vi "DiffDrivePoseEst2_Absolute_Example.vi"() -> ()   [LabVIEW 2019]
doc: "This WebSockets API example VI acts as a server for an incoming websockets connection. Receives/sends string data to the connected client."
uses:
  <vilib>/Rock Robotics/WPI/ThirdParty/JAS_Junk/TrajLib/Trajectory_Library.lvlib
  <vilib>/Rock Robotics/WPI/ThirdParty/JAS_Junk/TrajLib/TypeDef/FieldDisp_ElementPicture.ctl
  <vilib>/Rock Robotics/WPI/ThirdParty/JAS_Junk/TrajLib/TypeDef/TRANSLATION2D.ctl
  <vilib>/Rock Robotics/WPI/ThirdParty/JAS_Junk/TrajLib/TypeDef/ROTATION2D.ctl
  <vilib>/Rock Robotics/WPI/ThirdParty/JAS_Junk/TrajLib/TypeDef/POSE2D.ctl
panel:
  in  "Ramsette\nAuto":bool=TRUE
  out "Trajectory\nAtReference":bool
  out "ROBOT":T1
  in  "Tab Control":T2(tab)
  out "Field Picture":picture
  out "Right Motor Dmd":dbl format="%20.3f"
  out "Left Motor Dmd":dbl format="%20.3f"
  out "Gyro Heading (Deg)":dbl format="%20.3f"
  out "Left Motor Dist (Ft)":dbl format="%20.3f"
  out "Right Motor Dist (Ft)":dbl format="%20.3f"
  out "Left Motor Vel - PV (Ft/Sec)":dbl format="%20.3f"
  out "Right Motor Vel - PV (Ft/Sec)":dbl format="%20.3f"
  out "Odometry sim abs\n Pose SI":T3={"TRANSLATION"={"X"=1.0, "Y"=1.0}, "ROTATION"={"VALUE"=0.0, "COS"=1.0, "SIN"=0.0}} {"ROTATION"."SIN" format="%13.4f"; "ROTATION"."COS" format="%13.4f"; "ROTATION"."VALUE" format="%13.4f"; "TRANSLATION"."Y" format="%14.3f"; "TRANSLATION"."X" format="%14.3f"}
  out "Odom Abs Pose SI":T3 {"ROTATION"."SIN" format="%13.4f"; "ROTATION"."COS" format="%13.4f"; "ROTATION"."VALUE" format="%13.4f"; "TRANSLATION"."Y" format="%14.3f"; "TRANSLATION"."X" format="%14.3f"}
  out "Trajectory Error":T6(graph)
  in  "Follow Absolute\nTrajectory":bool
  in  "Spin Right":bool
  in  "Spin Left":bool
  in  "Reverse":bool
  in  "Forward":bool
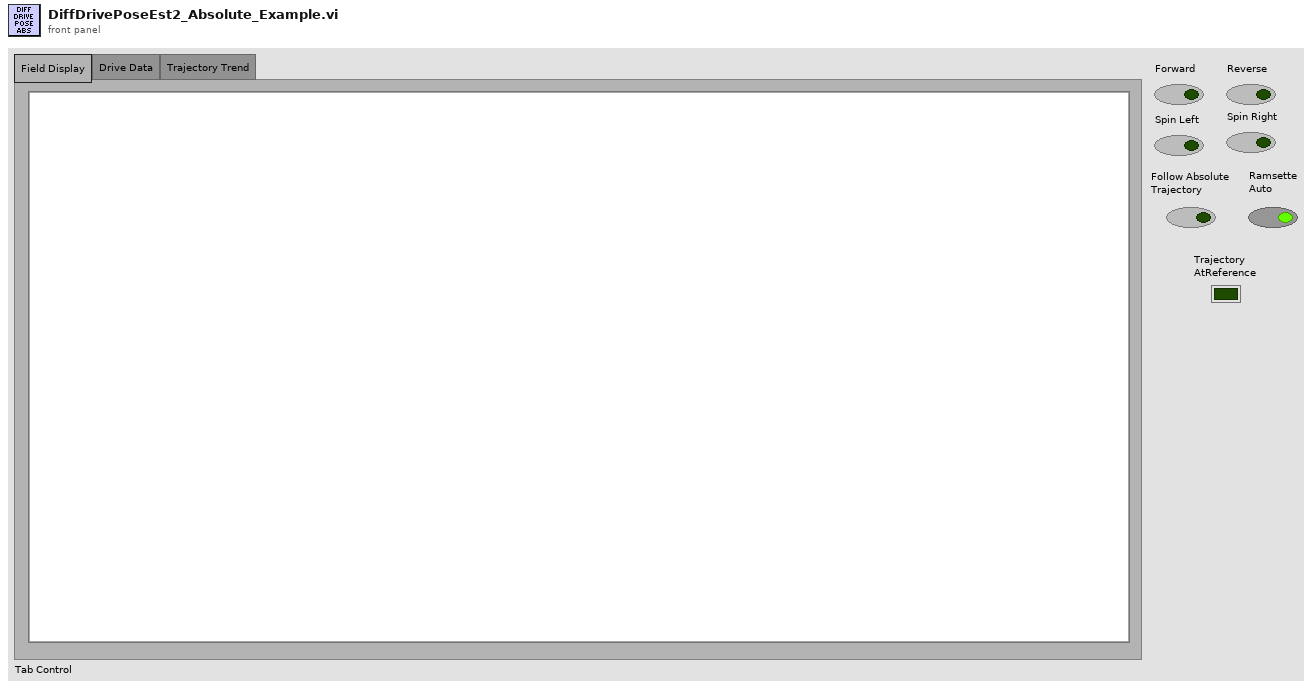
[diagram p1: front panel]
types:
  T1 = typedef "Trajectory_Library.lvlib/FieldDisp_ElementPicture.ctl" = picture
  T2 = enum32{"Field Display", "Drive Data", "Trajectory Trend"}
  T3 = typedef "Trajectory_Library.lvlib/POSE2D.ctl" = cluster{"TRANSLATION":T4, "ROTATION":T5}
  T4 = typedef "Trajectory_Library.lvlib/TRANSLATION2D.ctl" = cluster{"X":dbl, "Y":dbl}
  T5 = typedef "Trajectory_Library.lvlib/ROTATION2D.ctl" = cluster{"VALUE":dbl, "COS":dbl, "SIN":dbl}
  T6 = cluster{"Traj X Err Ft":dbl, "Traj Y Err Ft":dbl, "Traj Heading Err Deg":dbl, dbl}
  T7 = typedef "Trajectory_Library.lvlib/FieldDisp_FieldElement.ctl" = cluster{"ONE-8-bit pixmap":u8[][], "Two-Array":cdb[][], "Three-Numeric":i32, "Four-Numeric":i32, "Five-Numeric":cdb, "Six-colors":u32[], "Seven-new element/subarray":u32, "Left Poxel":dbl, "Top Pixel":dbl, "Width Pix/Ft":dbl, "Height Pix/Ft":dbl, "Element Picture Ref":refnum<vi>}
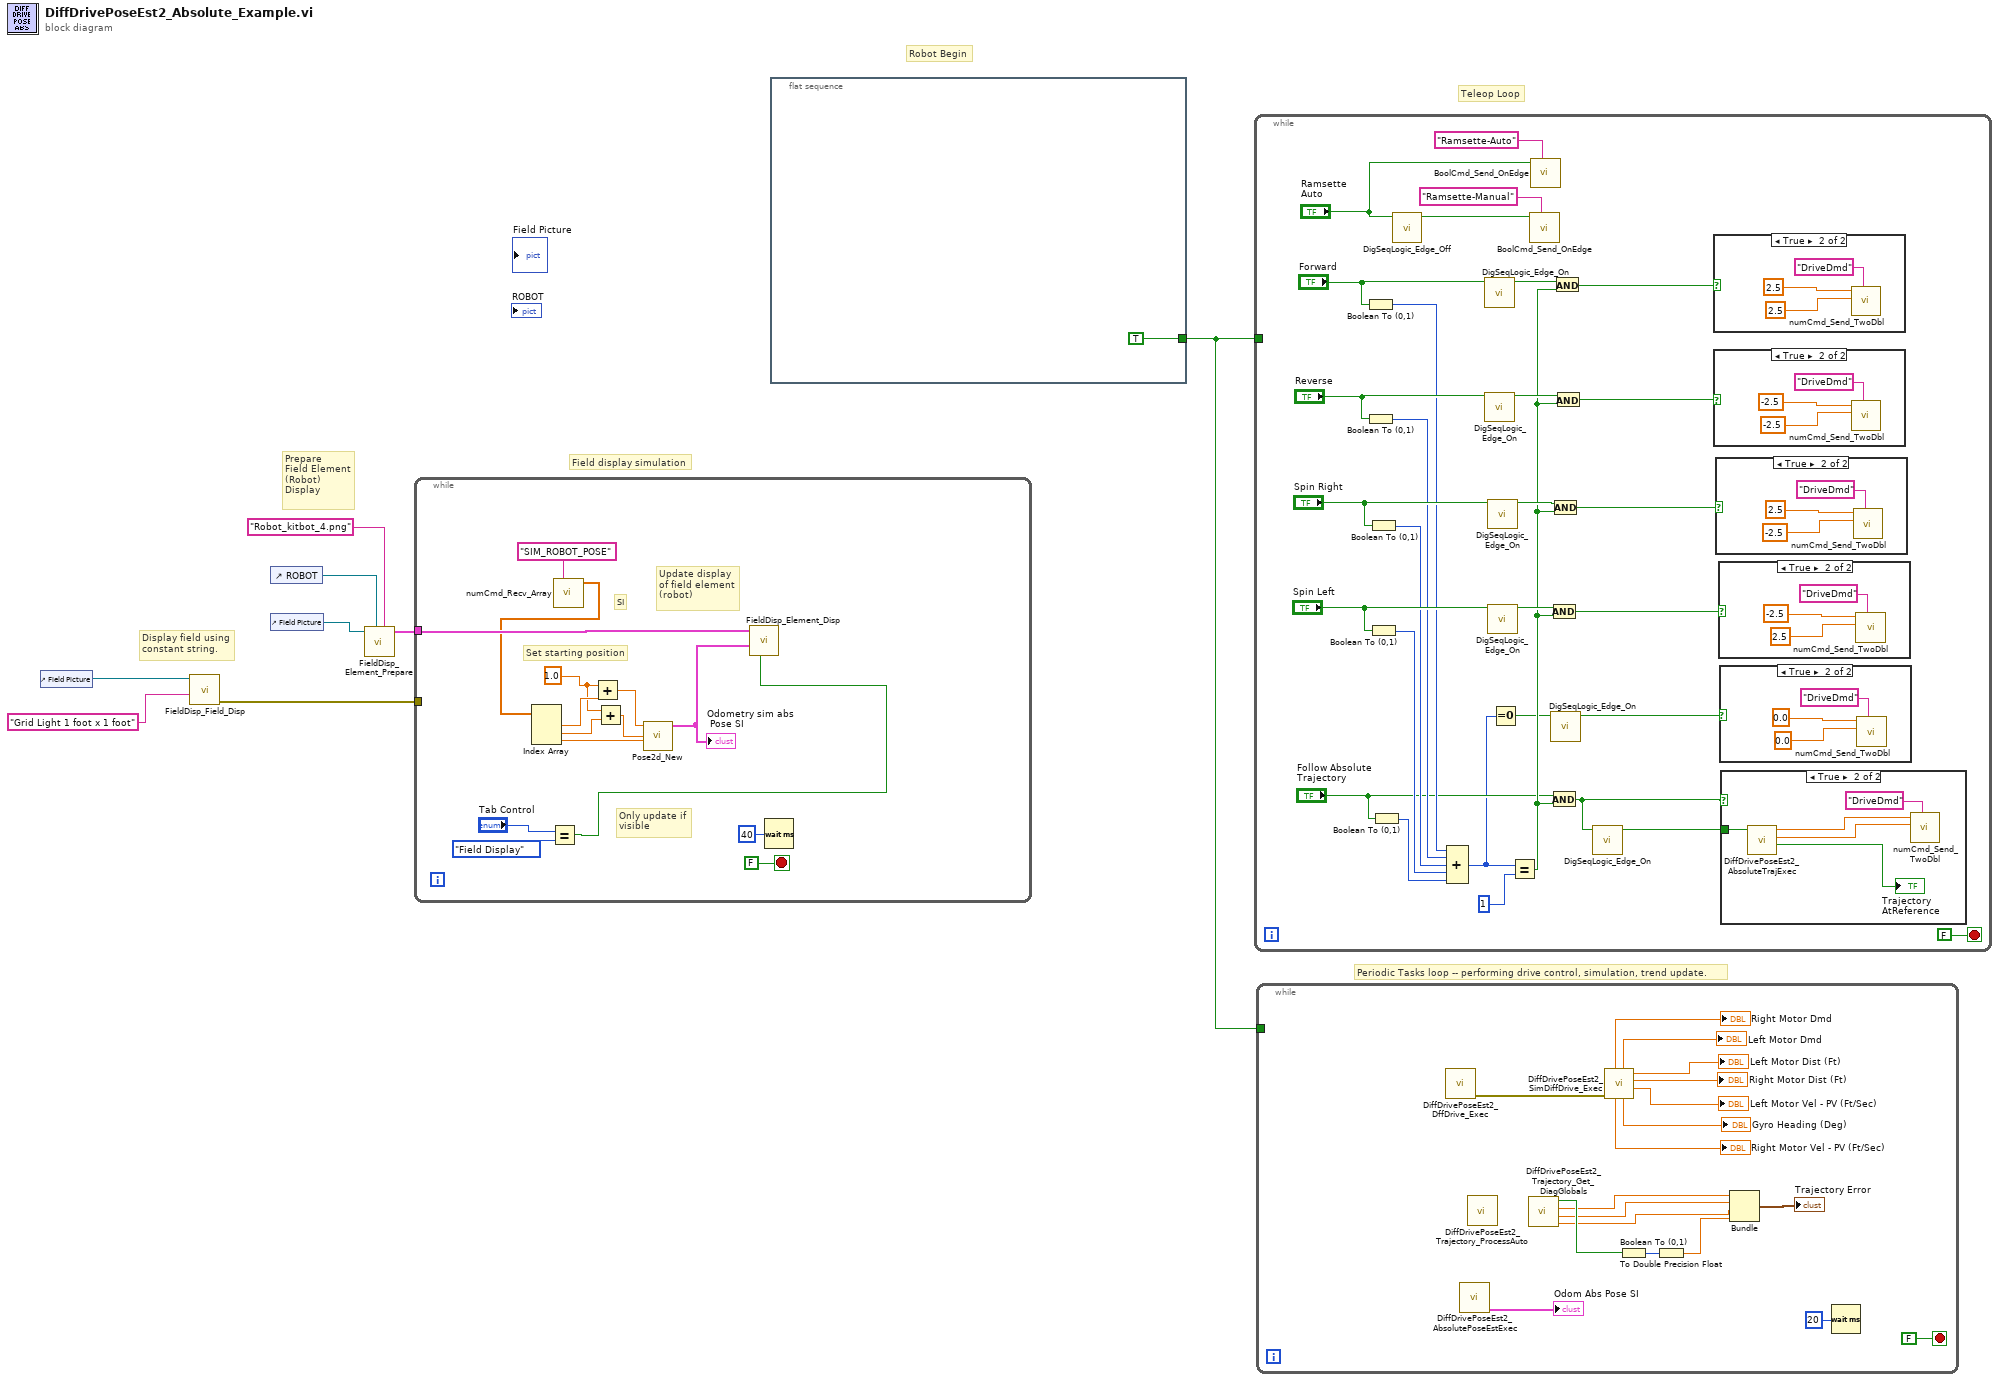
[diagram p0: block diagram]
diagram:
  # "Robot Begin"
  # "Periodic Tasks loop -- performing drive control, simulation, trend update."
  # "Field display simulation"
  # "Teleop Loop"
  # "Display field using\nconstant string."
  # "Prepare\nField Element\n(Robot)\nDisplay"
  n1 = control-ref of="Field Picture"() -> (w4:refnum<vi>)
  n2 = call <vilib>:"FieldDisp_Field_Disp.vi"("Field Selector"="Grid Light 1 foot x 1 foot", "Picture in"=w4) -> ("error out"=w2:errorcluster)  [unwired: 9 in]
  n3 = control-ref of="ROBOT"() -> (w7:refnum<vi>)
  n4 = control-ref of="Field Picture"() -> (w8:refnum<vi>)
  n5 = call <vilib>:"FieldDisp_Element_Prepare.vi"("Element File Name"="Robot_kitbot_4.png" ("Picture FIle Name"), "Element Picture Ref"=w7, "Field Picture Ref"=w8) -> ("Field Element Info"=w5:T7)  [unwired: 7 in, 1 out]
  n6 = while {
    tunnel: w5 -> [w21]
    tunnel: w2 -> [_]
    stop <- FALSE stop-if-true
    w10 = 1.0 ("x")
    # "SI"
    # "Set starting position"
    # "Update display\nof field element\n(robot)"
    # "Only update if\nvisible"
    n7 = Equal?(x="Tab Control", y=T2."Field Display") -> (x = y?=w9:bool)
    n8 = call <vilib>:"numCmd_Recv_Array.vi"("Command Name"="SIM_ROBOT_POSE") -> ("Values"=w17:dbl[])  [unwired: 8 in, 2 out]
    n9 = Index Array(array=w17) -> (element #1=w11:dbl, element #2=w12:dbl, element #3=w16:dbl)  [unwired: 3 in]
    n10 = Add(x=w10, y=w11) -> (x+y=w13:dbl)
    n11 = Add(x=w10, y=w12) -> (x+y=w14:dbl)
    n12 = call <vilib>:"Pose2d_New.vi"("Heading"=w16, "Y"=w14, "X"=w13) -> ("out POSe"=w15:T3)  [unwired: 8 in]
    "Odometry sim abs\n Pose SI" <- w15
    n13 = call <vilib>:"FieldDisp_Element_Disp.vi"("Visible"=w9, "Element Pose"=w15, "Element Info"=w21) -> ()  [unwired: 9 in]
    n14 = Wait (ms)(milliseconds to wait=u32 40) -> ()  [unwired: 1 out]
  }
  n15 = flat-sequence {
    tunnel: [TRUE] -> w1
    frame #0 {
    }
  }
  n16 = while {
    tunnel: w1 -> [_]
    stop <- FALSE stop-if-true
    n17 = Boolean To (0,1)(Boolean="Forward") -> (0, 1=w46:i16)
    n18 = Boolean To (0,1)(Boolean="Reverse") -> (0, 1=w47:i16)
    n19 = Boolean To (0,1)(Boolean="Spin Right") -> (0, 1=w48:i16)
    n20 = Boolean To (0,1)(Boolean="Spin Left") -> (0, 1=w49:i16)
    n21 = Boolean To (0,1)(Boolean="Follow Absolute\nTrajectory") -> (0, 1=w50:i16)
    n22 = call <vilib>:"DigSeqLogic_Edge_Off.vi"("Input"="Ramsette\nAuto") -> ("Off Edge"=w27:bool)  [unwired: 10 in]
    n23 = Compound Arithmetic op=ADD(w46, w47, w48, w49, w50) -> (w38:i16)
    n24 = call <vilib>:"DigSeqLogic_Edge_On.vi"("Input"="Forward") -> ("On Edge"=w44:bool)  [unwired: 10 in]
    n25 = call <vilib>:"DigSeqLogic_Edge_On.vi"("Input"="Reverse") -> ("On Edge"=w43:bool)  [unwired: 10 in]
    n26 = call <vilib>:"DigSeqLogic_Edge_On.vi"("Input"="Spin Right") -> ("On Edge"=w42:bool)  [unwired: 10 in]
    n27 = call <vilib>:"DigSeqLogic_Edge_On.vi"("Input"="Spin Left") -> ("On Edge"=w41:bool)  [unwired: 10 in]
    n28 = Equal To 0?(x=w38) -> (x = 0?=w37:bool)
    n29 = Equal?(x=w38, y=i16 1) -> (x = y?=w40:bool)
    n30 = call <vilib>:"BoolCmd_Send_OnEdge.vi"("Command Name"="Ramsette-Manual", "Value"=w27) -> ()  [unwired: 9 in, 1 out]
    n31 = call <vilib>:"BoolCmd_Send_OnEdge.vi"("Command Name"="Ramsette-Auto", "Value"="Ramsette\nAuto") -> ()  [unwired: 9 in, 1 out]
    n32 = And(x=w41, y=w40) -> (x .and. y?=w32:bool)
    n33 = And(x="Follow Absolute\nTrajectory", y=w40) -> (x .and. y?=w31:bool)
    n34 = And(x=w42, y=w40) -> (x .and. y?=w34:bool)
    n35 = call <vilib>:"DigSeqLogic_Edge_On.vi"("Input"=w37) -> ("On Edge"=w33:bool)  [unwired: 10 in]
    n36 = And(x=w44, y=w40) -> (x .and. y?=w36:bool)
    n37 = And(x=w43, y=w40) -> (x .and. y?=w35:bool)
    n38 = call <vilib>:"DigSeqLogic_Edge_On.vi"("Input"=w31) -> ("On Edge"=w30:bool)  [unwired: 10 in]
    n39 = case shown="True" w36 {
      frame False {
      }
      frame True {
        n40 = call <vilib>:"numCmd_Send_TwoDbl.vi"("Command Name"="DriveDmd", "Value 2"=2.5, "Value 1"=2.5) -> ()  [unwired: 8 in, 1 out]
      }
    }
    n41 = case shown="True" w35 {
      frame False {
      }
      frame True {
        n42 = call <vilib>:"numCmd_Send_TwoDbl.vi"("Command Name"="DriveDmd", "Value 2"=-2.5, "Value 1"=-2.5) -> ()  [unwired: 8 in, 1 out]
      }
    }
    n43 = case shown="True" w34 {
      frame False {
      }
      frame True {
        n44 = call <vilib>:"numCmd_Send_TwoDbl.vi"("Command Name"="DriveDmd", "Value 2"=-2.5, "Value 1"=2.5) -> ()  [unwired: 8 in, 1 out]
      }
    }
    n45 = case shown="True" w32 {
      frame False {
      }
      frame True {
        n46 = call <vilib>:"numCmd_Send_TwoDbl.vi"("Command Name"="DriveDmd", "Value 2"=2.5, "Value 1"=-2.5) -> ()  [unwired: 8 in, 1 out]
      }
    }
    n47 = case shown="True" w33 {
      frame False {
      }
      frame True {
        n48 = call <vilib>:"numCmd_Send_TwoDbl.vi"("Command Name"="DriveDmd", "Value 2"=0.0, "Value 1"=0.0) -> ()  [unwired: 8 in, 1 out]
      }
    }
    n49 = case shown="True" w31 {
      tunnel: w30 -> [_ w55]
      frame False {
      }
      frame True {
        n50 = call "DiffDrivePoseEst2_AbsoluteTrajExec.vi"("Init"=w55) -> ("AtReference"=→"Trajectory\nAtReference":bool, "Right Speed Target"=w57:dbl, "Left Speed Target"=w58:dbl)  [unwired: 7 in, 1 out]
        n51 = call <vilib>:"numCmd_Send_TwoDbl.vi"("Command Name"="DriveDmd", "Value 2"=w57, "Value 1"=w58) -> ()  [unwired: 8 in, 1 out]
      }
    }
  }
  n52 = while {
    tunnel: w1 -> [_]
    stop <- FALSE stop-if-true
    n53 = call "DiffDrivePoseEst2_DffDrive_Exec.vi"() -> ("error out"=w83:errorcluster)  [unwired: 11 in]
    n54 = call "DiffDrivePoseEst2_AbsolutePoseEstExec.vi"() -> ("Abs Pose Est SI"=→"Odom Abs Pose SI":T3)  [unwired: 11 in]
    n55 = call "DiffDrivePoseEst2_Trajectory_ProcessAuto.vi"() -> ()  [unwired: 12 in]
    n56 = call "DiffDrivePoseEst2_Trajectory_Get_DiagGlobals.vi"() -> ("Traj Heading Err Deg"=w76:dbl, "Traj Y Err Ft"=w77:dbl, "Traj X Err Ft"=w78:dbl, "AtReference"=w80:bool)  [unwired: 8 in]
    n57 = call "DiffDrivePoseEst2_SimDiffDrive_Exec.vi"("error in (no error)"=w83) -> ("Left Motor Vel - PV (Ft/Sec)"=→"Left Motor Vel - PV (Ft/Sec)":dbl, "Right Motor Dist (Ft)"=→"Right Motor Dist (Ft)":dbl, "Left Motor Dist (Ft)"=→"Left Motor Dist (Ft)":dbl, "Gyro Heading (Deg)"=→"Gyro Heading (Deg)":dbl, "Left Motor Dmd"=→"Left Motor Dmd":dbl, "Right Motor Vel - PV (Ft/Sec)"=→"Right Motor Vel - PV (Ft/Sec)":dbl, "Right Motor Dmd"=→"Right Motor Dmd":dbl)  [unwired: 3 in, 1 out]
    n58 = Boolean To (0,1)(Boolean=w80) -> (0, 1=w81:i16)
    n59 = To Double Precision Float(number=w81) -> (double precision float=w79:dbl)
    n60 = Bundle("Traj X Err Ft"=w78, "Traj Y Err Ft"=w77, "Traj Heading Err Deg"=w76, w79) -> (→"Trajectory Error":T6)  [unwired: 1 in]
    n61 = Wait (ms)(milliseconds to wait=u32 20) -> ()  [unwired: 1 out]
  }
